vi "Filter circles.vi"(0 "Circ x":dbl[](array[numeric]), 1 "Circ y":dbl[](array[numeric]), 2 "R":dbl[](array[numeric]), 3 "LRF pos":dbl[](array[numeric]), 4 "max dist":dbl) -> (5 "Circ x out":dbl[](array[numeric]), 6 "Circ y out":dbl[](array[numeric]), 7 "R out":dbl[](array[numeric]))   [LabVIEW 2009]
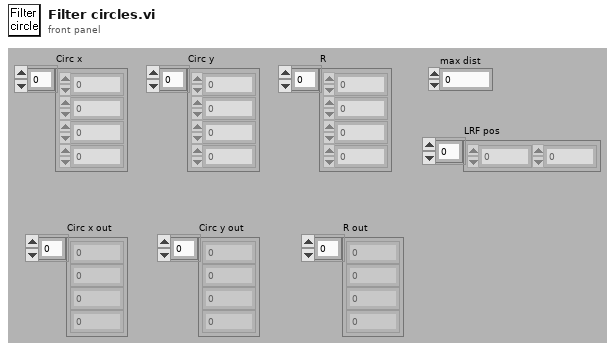
[diagram p1: front panel]
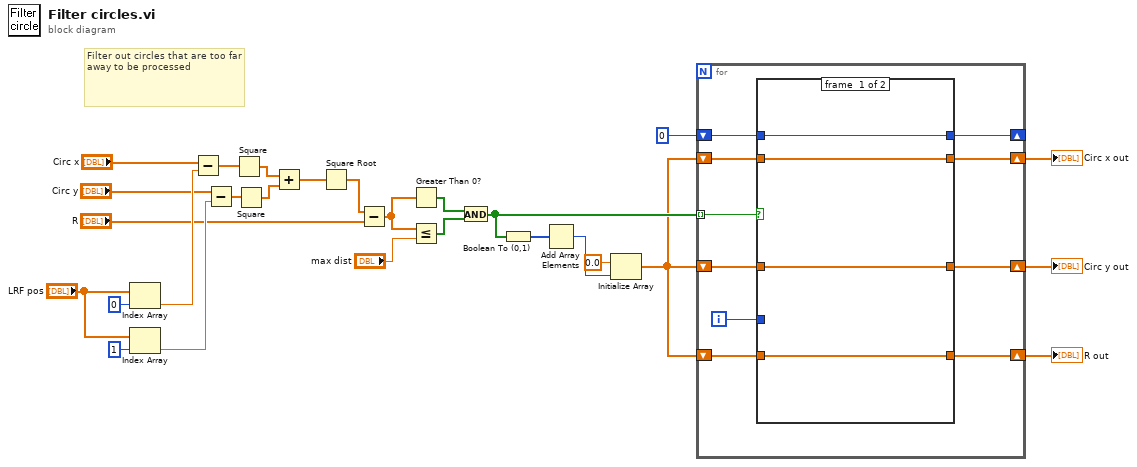
[diagram p0: block diagram]
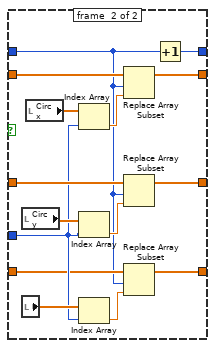
[diagram p2: hidden frame]
diagram:
  # "Filter out circles that are too far away to be processed"
  n1 = Index Array(array="LRF pos", index=0) -> (element=w23:dbl)
  n2 = Index Array(array="LRF pos", index=1) -> (element=w21:dbl)
  n3 = Subtract(x="Circ x", y=w23) -> (x-y=w20:dbl[])
  n4 = Subtract(x="Circ y", y=w21) -> (x-y=w19:dbl[])
  n5 = Square(x=w20) -> (x^2=w18:dbl[])
  n6 = Square(x=w19) -> (x^2=w17:dbl[])
  n7 = Add(x=w18, y=w17) -> (x+y=w16:dbl[])
  n8 = Square Root(x=w16) -> (sqrt(x)=w15:dbl[])
  n9 = Subtract(x=w15, y="R") -> (x-y=w12:dbl[])
  n10 = Greater Than 0?(x=w12) -> (x > 0?=w11:bool[])
  n11 = Less Or Equal?(x=w12, y="max dist") -> (x <= y?=w10:bool[])
  n12 = And(x=w11, y=w10) -> (x .and. y?=w9:bool[])
  n13 = Boolean To (0,1)(Boolean=w9) -> (0, 1=w8:i16[])
  n14 = Add Array Elements(numeric array=w8) -> (sum=w7:i16)
  n15 = Initialize Array(0.0 ("element"), w7) -> (w5:dbl[])
  n16 = for {
    tunnel: w9 -> [w37] mode=indexing
    shift-right: [w30] -> w2
    shift-left: w5 -> [w31]
    shift-right: [w33] -> w3
    shift-left: w5 -> [w36]
    shift-right: [w29] -> w1
    shift-left: w5 -> [w28]
    shift-right: [w34] -> _
    shift-left: 0 -> [w35]
    i -> [w32]
    n17 = case shown="True" w37 {
      tunnel: w36 -> [w40 w56]
      tunnel: w35 -> [w41 w42]
      tunnel: [w41 w54] -> w34
      tunnel: [w40 w52] -> w33
      tunnel: w32 -> [_ w45]
      tunnel: w31 -> [w39 w48]
      tunnel: [w39 w47] -> w30
      tunnel: [w38 w43] -> w29
      tunnel: w28 -> [w38 w44]
      frame #0 {
      }
      frame #1 {
        n18 = local read "Circ y"() -> (w49:dbl[])
        n19 = local read "R"() -> (w46:dbl[])
        n20 = local read "Circ x"() -> (w55:dbl[])
        n21 = Index Array(array=w55, index=w45) -> (element=w53:dbl)
        n22 = Index Array(array=w49, index=w45) -> (element=w51:dbl)
        n23 = Index Array(array=w46, index=w45) -> (element=w50:dbl)
        n24 = Replace Array Subset(array=w56, new element=w53, index=w42) -> (w52:dbl[])
        n25 = Replace Array Subset(array=w48, new element=w51, index=w42) -> (w47:dbl[])
        n26 = Replace Array Subset(array=w44, new element=w50, index=w42) -> (w43:dbl[])
        n27 = Increment(x=w42) -> (x+1=w54:i32)
      }
    }
  }
  "Circ x out" <- w3
  "Circ y out" <- w2
  "R out" <- w1
